vi "Uint16 Destroy.vi"(8 "error in (no error)":errorcluster, 11 "Uint16 DVR in":refnum<data-value>) -> (0 "error out":errorcluster)   [LabVIEW 2012, in "MDSplus.lvlib"]
uses:
  <vilib>/MDSplus/Library/MDSplus.lvlib
  <vilib>/MDSplus/Classes/Data_Class/Scalar_Class/Uint16_Class/Uint16.lvclass
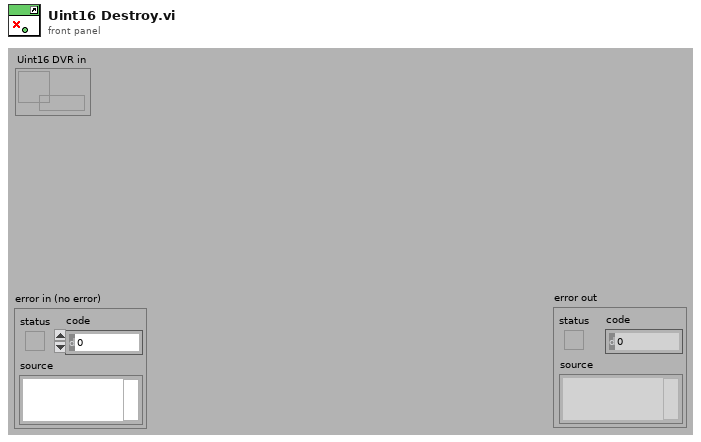
[diagram p1: front panel]
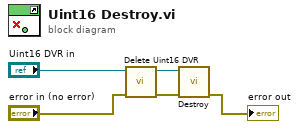
[diagram p0: block diagram]
diagram:
  n1 = call <vilib>:"Delete Uint16 DVR.vi"("error in (no error)"="error in (no error)", "Uint16 DVR in"="Uint16 DVR in") -> ("error out"=w2:errorcluster, "Uint16 out"=w3:refnum<class "Uint16.lvclass">)  [unwired: 8 in]
  n2 = call-dynamic "Destroy.vi"("error in (no error)"=w2, "Uint16 in"=w3) -> ("error out"=→"error out":errorcluster)  [unwired: 9 in]
